vi "HXG2_TC1-8_Strings_FGV.vi"(7 "GraphScales":T1, 8 "error in (no error)":errorcluster, 11 "TCs1-8Strings In":string[](array[string])) -> (0 "error out":errorcluster, 3 "TCs1-8Strings Out":string[](array[string]))   [LabVIEW 2010]
uses:
  HXG2graphscales.ctl
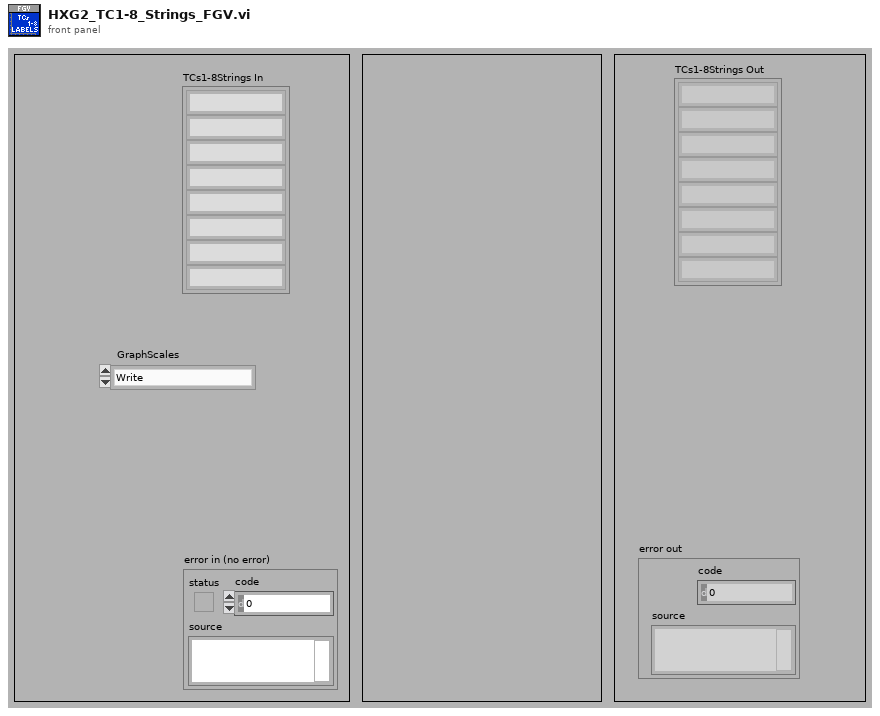
[diagram p1: front panel]
types:
  T1 = typedef "HXG2graphscales.ctl" = enum16{"Write", "Pass"}
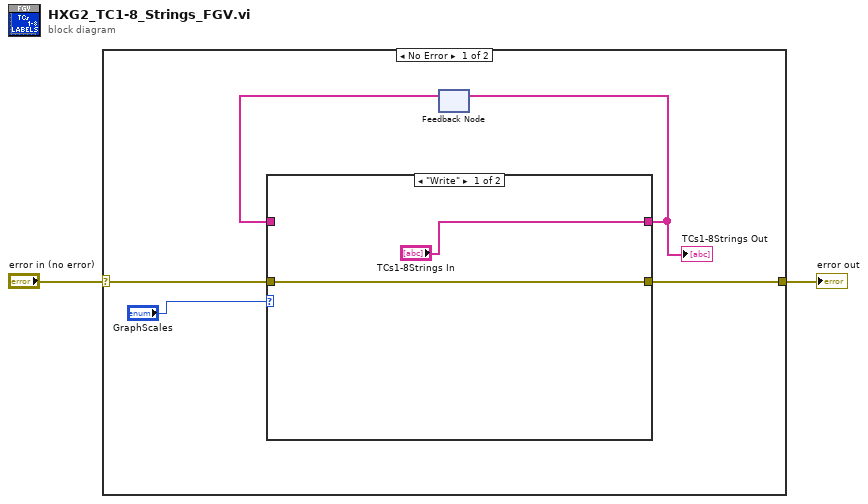
[diagram p0: block diagram]
diagram:
  n1 = case shown="No Error" "error in (no error)" {
    selector: "error in (no error)" -> [w7 w12]
    tunnel: [w6 w12] -> w1
    frame No Error {
      n2 = feedback #1() -> (w5:string[])  [unwired: 1 in]
      n3 = case shown="\"Write\"" "GraphScales" {
        tunnel: w7 -> [w9 w10]
        tunnel: [w9 w10] -> w6
        tunnel: ["TCs1-8Strings In" w11] -> w3
        tunnel: w5 -> [_ w11]
        frame "Write" {
        }
        frame "Pass" {
        }
      }
      "TCs1-8Strings Out" <- w3
      n4 = feedback-in #1(w3) -> ()
    }
    frame Error {
    }
  }
  "error out" <- w1
